vi "database_update.vi"(8 "error in (no error)":errorcluster, 11 "path to csv file":path) -> ()   [LabVIEW 2017]
uses:
  <vilib>/Utility/file.llb/Read Delimited Spreadsheet (string).vi
  <vilib>/Utility/file.llb/Write Delimited Spreadsheet (string).vi
panel:
  out "output array":string[](array[string])
  in  "file path (dialog if empty)":path=path "C:/Users/Lenovo/Desktop/szakdoga/data/database.csv"
  out "all rows":string[][](array[string])
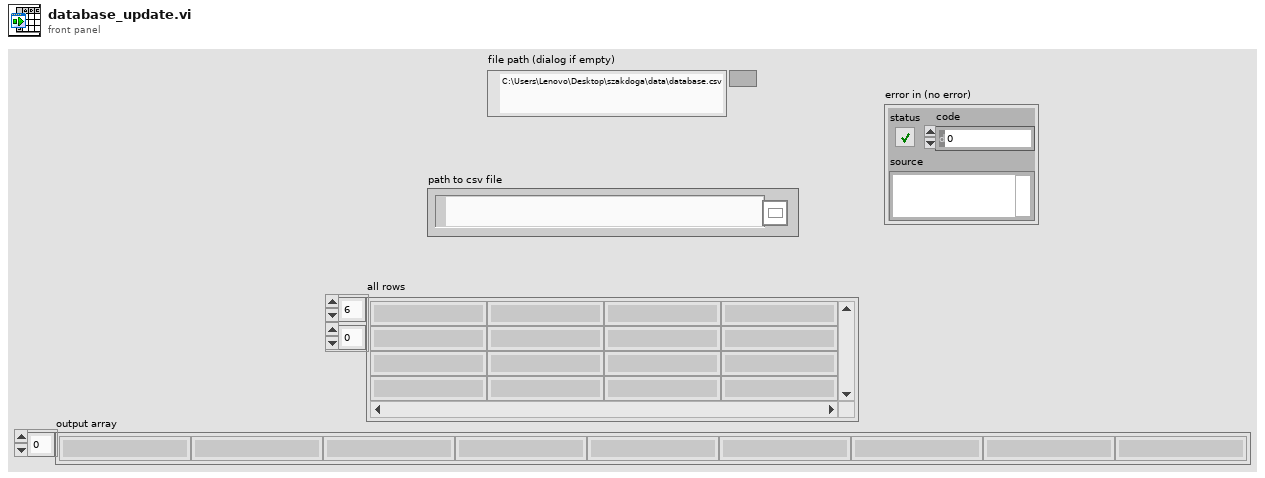
[diagram p1: front panel]
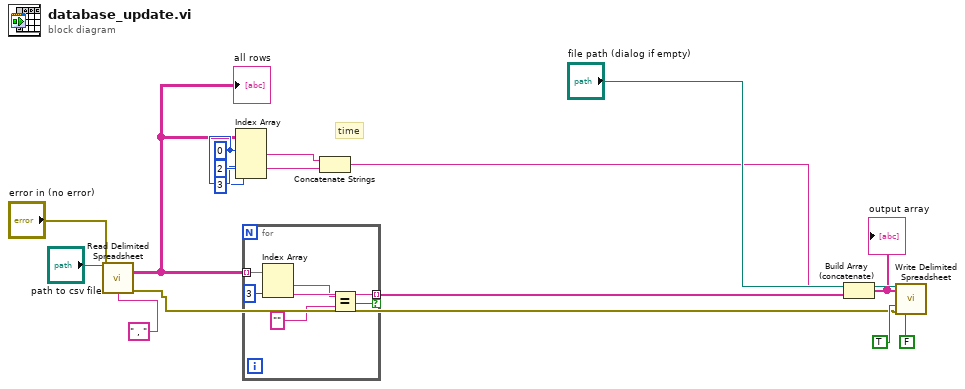
[diagram p0: block diagram]
diagram:
  w8 = 0 ("index (row)")
  # "time"
  n1 = call-poly <vilib>:"Read Delimited Spreadsheet.vi"("file path (dialog if empty)"="path to csv file", "error in (no error)"="error in (no error)", "delimiter (\\t)"=" , " ("delimiter (\\t)")) -> ("all rows"=w3:string[][], "error out"=w12:errorcluster)  [unwired: 7 in, 4 out]
  "all rows" <- w3
  n2 = Index Array(array=w3, index (row) #1=w8, index (col) #1=2 ("disabled index (col)"), index (row) #2=w8, index (col) #2=3 ("disabled index (col)")) -> (element #1=w6:string, element #2=w5:string)
  n3 = for {
    tunnel: w3 -> [w22] mode=indexing
    tunnel: [w21] -> w2 mode=indexing if=w20
    n4 = Index Array(array=w22, index #2=3 ("index")) -> (element #1=w18:string, element #2=w21:string)  [unwired: 1 in]
    n5 = Equal?(x=w18, y="") -> (x = y?=w20:bool)
  }
  n6 = Concatenate Strings(w6, w5) -> (w4:string)
  n7 = Build Array (concatenate)(w4, w2) -> (w9:string[])
  "output array" <- w9
  n8 = call-poly <vilib>:"Write Delimited Spreadsheet.vi"("file path (dialog if empty)"="file path (dialog if empty)", "1D data"=w9, "append to file? (new file:F)"=TRUE, "error in (no error)"=w12, "transpose? (no:F)"=FALSE) -> ()  [unwired: 9 in, 2 out]
